vi "Build Actual Engine Group.vi"(8 "error in (no error)":errorcluster, 11 "Device Item Ref in":T1 format="%.0x") -> (0 "error out":errorcluster, 2 "Group":T2 {"VS Refs" format="%.0x"}, 3 "Section Ref out":T1 format="%.0x")   [LabVIEW 2017, in "NI 272x Resistive Simulation Custom Device Configuration.lvlib"]
uses:
  NI 272x Resistive Simulation Custom Device Configuration.lvlib
  <vilib>/NI Veristand/Custom Device API/Custom Device Item Ref.ctl
  <vilib>/NI Veristand/Custom Device Tools/Custom Device Utility Library/NI VeriStand - Search for Item by Name.vi
  Globals/Names.vi
  <vilib>/NI VeriStand/Custom Device Tools/Custom Device Utility Library/Custom Device Utility Library.lvlib
  <vilib>/NI VeriStand/Custom Device API/Custom Device API.lvlib
  NI 272x Resistive Simulation Custom Device Shared.lvlib
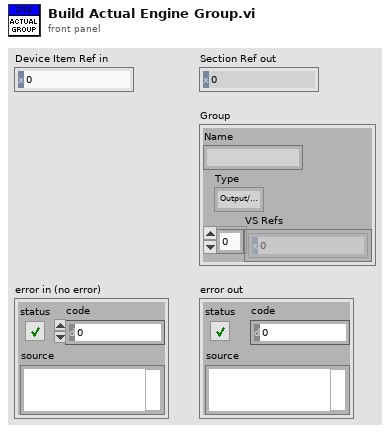
[diagram p1: front panel]
types:
  T1 = typedef "Custom Device API.lvlib/Custom Device Item Ref.ctl" = u64
  T2 = cluster{"Name":string, "Type":enum16{"Output/Write", "Input/Read", "Input/ReadWrite"}, "VS Refs":T1[]}
  T3 = enum16{"Output/Write", "Input/Read", "Input/ReadWrite"}
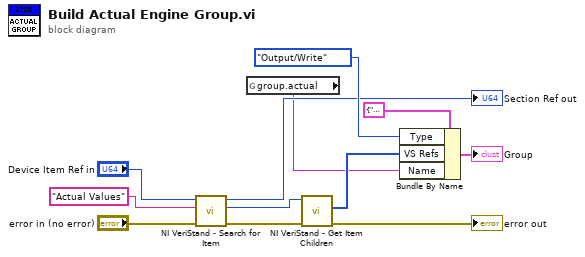
[diagram p0: block diagram]
diagram:
  n1 = call-poly <vilib>:"NI VeriStand - Search for Item.vi"("error in"="error in (no error)", "Item Name"="Actual Values", "Section Ref in"="Device Item Ref in") -> ("error out"=w3:errorcluster, "Item Ref"=w7:T1, "Section Ref out"=→"Section Ref out":T1)  [unwired: 5 in, 1 out]
  n2 = global read "Names.vi" "group.actual"() -> (w1:string)
  n3 = call <vilib>:"NI VeriStand - Get Item Children.vi"("error in (no error)"=w3, "Item Ref in"=w7) -> ("error out"=→"error out":errorcluster, "Child Refs"=w11:T1[])  [unwired: 6 in, 2 out]
  n4 = Bundle By Name(cluster=T2 {"Name"="", "Type"=enum."Output/Write", "VS Refs"=[]} ("Group"), "Type"=T3."Output/Write", "VS Refs"=w11, "Name"=w1) -> (→"Group":T2)
